vi "Load Default Configuration.vi"(8 "error in (no error)":errorcluster, 11 "CIFPlugin in":refnum<class "Template_Plugin.lvclass">) -> (0 "error out":errorcluster, 3 "CIFPlugin out":refnum<class "Template_Plugin.lvclass">)   [LabVIEW 2021, in "Template_Plugin.lvclass"]
uses:
  Template_Plugin.lvclass
  C:/Program Files/National Instruments/LabVIEW 2021/vi.lib/CIF Foundation/CIF Core/CIFCore/Class/CIFCorePlugin.lvclass
  <vilib>/CIF Foundation/CIF Core/CIFCore/Common/Typedef/Common Plugin Configuration.ctl
  Template_Plugin.lvclass/Template_Plugin.ctl
  <vilib>/CIF Foundation/CIF Core/CIFCore/Class/CIFCorePlugin.lvclass/CIFCorePlugin.ctl
  <vilib>/CIF Foundation/CIF Core/CIFCore/Class/SubVIs/OOB/Send/Load Payload.vi
  <vilib>/CIF Foundation/CIF Core/CIFCore/Class/Accessors/Read Plugin Name.vi
  <vilib>/CIF Foundation/CIF Core/CIFCore/Class/Accessors/Read Version.vi
  <vilib>/CIF Foundation/CIF Core/CIFUtilities/CIFLogs/Utilities/Create Version String.vi
  <vilib>/addons/_JKI.lib/Serialization/JSON/Library/Flatten To JSON String.vi
  <vilib>/CIF Foundation/CIF Core/CIFUtilities/CIFLogs/Utilities/Create JSON Config String.vi
  <vilib>/Utility/LVClass/Get LV Class Name.vi
  <vilib>/CIF Foundation/CIF Core/CIFUtilities/CIFLogs/Logs/Write to Config.vi
  <vilib>/CIF Foundation/CIF Core/CIFCore/Common/CIFCoreCommon.lvlib
  <vilib>/CIF Foundation/CIF Core/CIFCore/Class/CIFCorePlugin.lvclass
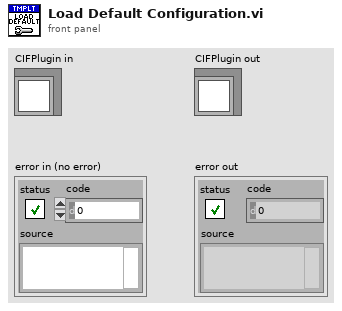
[diagram p1: front panel]
types:
  T1 = typedef "CIFCoreCommon.lvlib/Common Plugin Configuration.ctl" = cluster{"Period (s)":dbl, "Offset (us)":i32, "ClockID":u8, "Priority":i32, "Processor":i32}
  T2 = typedef "Template_Common.lvlib/Configuration.ctl" = cluster{"Common":T1, "Step":u64}
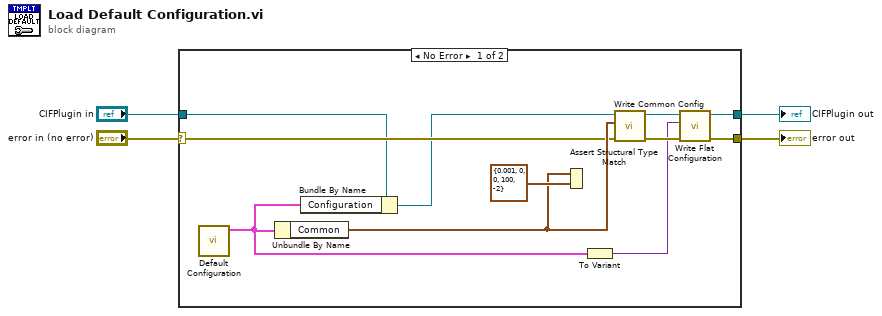
[diagram p0: block diagram]
diagram:
  n1 = case shown="No Error" "error in (no error)" {
    selector: "error in (no error)" -> [w8 w16]
    tunnel: "CIFPlugin in" -> [w7 w17]
    tunnel: [w11 w17] -> w1
    tunnel: [w10 w16] -> w3
    frame No Error {
      n2 = call "Default Configuration.vi"() -> ("Default Configuration"=w6:T2)  [unwired: 11 in]
      n3 = Unbundle By Name(w6) -> ("Common"=w14:T1)
      n4 = Bundle By Name(cluster=w7, "Configuration"=w6) -> (w5:refnum<class "Template_Plugin.lvclass">)
      n5 = Assert Structural Type Match(0:T1 {"Period (s)"=0.001, "Offset (us)"=0, "ClockID"=0, "Priority"=100, "Processor"=-2} ("Common"), 1:w14) -> ()
      n6 = To Variant(anything=w6) -> (Variant=w9:variant)
      n7 = call <vilib>:"Write Common Config.vi"("error in (no error)"=w8, "Common"=w14, "CIFTemplateNode in"=w5) -> ("error out"=w12:errorcluster, "CIFTemplateNode out"=w13:refnum<class "Template_Plugin.lvclass">)  [unwired: 7 in]
      n8 = call <vilib>:"Write Flat Configuration.vi"("error in (no error)"=w12, "Configuration"=w9, "CIFTemplateNode in"=w13) -> ("error out"=w10:errorcluster, "CIFTemplateNode out"=w11:refnum<class "Template_Plugin.lvclass">)  [unwired: 7 in]
    }
    frame Error {
    }
  }
  "error out" <- w3
  "CIFPlugin out" <- w1
